vi "WhichRobotGlobalVariable.vi"() -> ()   [LabVIEW 2011]
panel:
  out "Which robot are we using?":i16
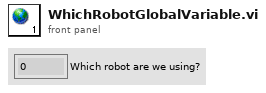
[diagram p1: front panel]
diagram:
